vi "skippable_AlliGator SS2 Dataset Load Option Dialog.vi"(8 "Error In":errorcluster) -> (0 "Error Out":errorcluster, 3 "SS2 8-bit Frame Selection":T1 caption="SS2 Frame Selection")   [LabVIEW 2021, in "AlliGator Files.lvlib"]
doc: "Skippable dialog to determine which 8-bit frame to load out of the 4 constituting a 10-bit dataset."
uses:
  AlliGator/AlliGator Files.lvlib
  SwissSPAD 8-bit Frames Read.ctl
  <vilib>/Utility/error.llb/Error Cluster From Error Code.vi
  <vilib>/ErrorRing/Error Ring.xnode
  AlliGator/AlliGator GUI.lvlib
  SwissSPAD.lvlib
panel:
  in  "Cancel":bool
  in  "SS2 Frame Selection":T1
  in  "OK":bool
  in  "Do not show this dialog again":bool
  out "Displayed Message":string="Select which 8-bit component to include in the final dataset:"
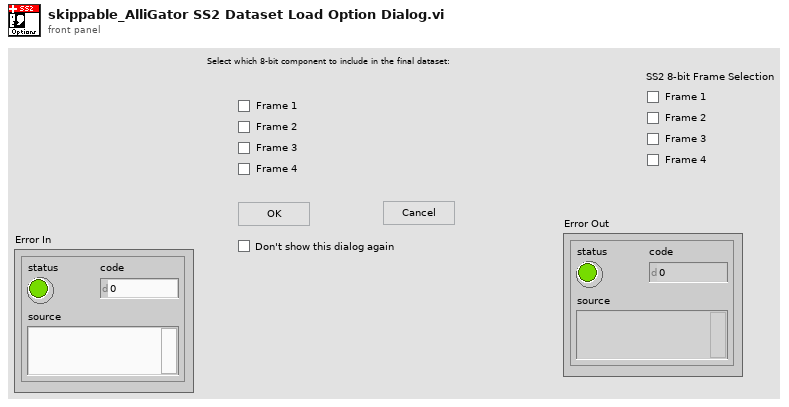
[diagram p1: front panel]
types:
  T1 = typedef "SwissSPAD.lvlib/SwissSPAD 8-bit Frames Read.ctl" = cluster{"Frame 1":bool, "Frame 2":bool, "Frame 3":bool, "Frame 4":bool}
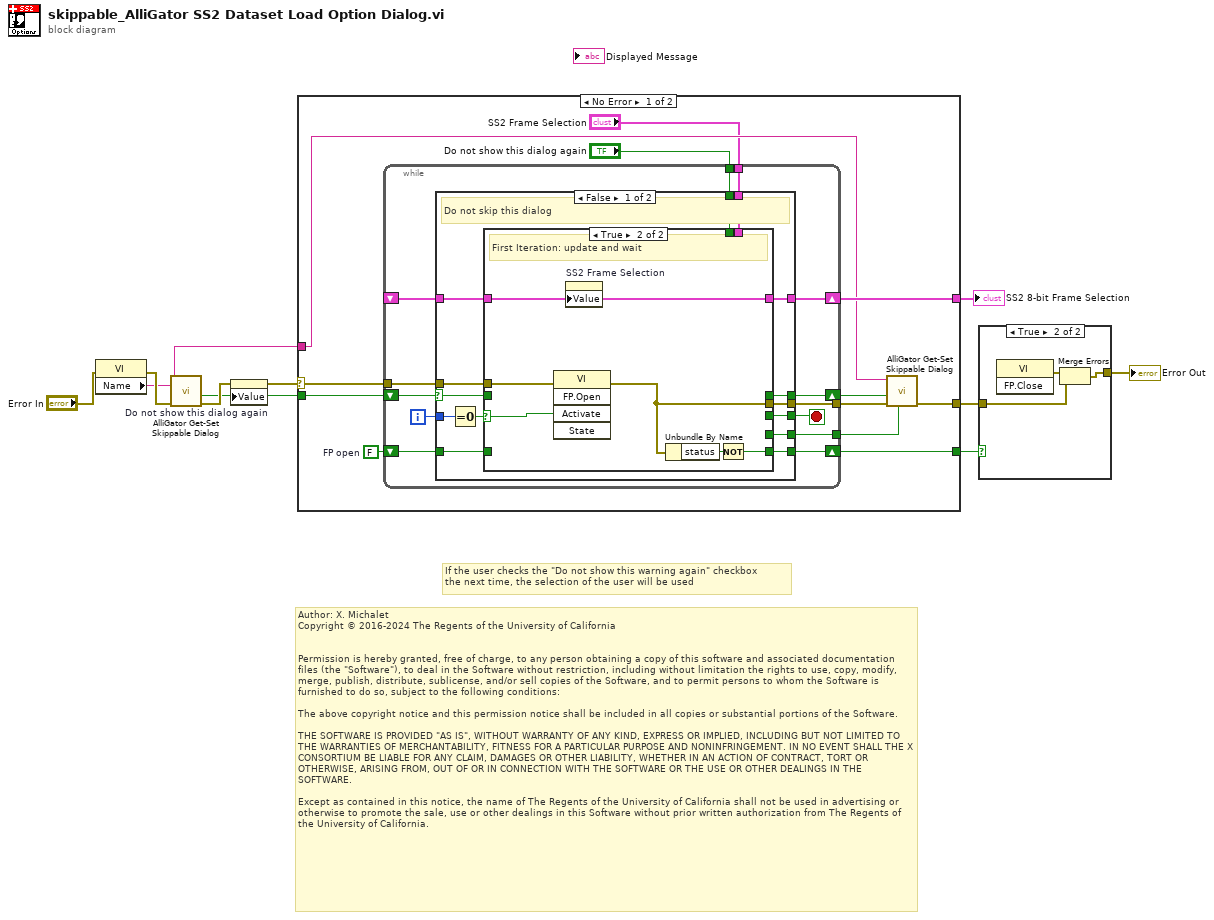
[diagram p0: block diagram]
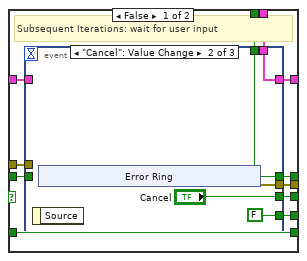
[diagram p3: hidden frame]
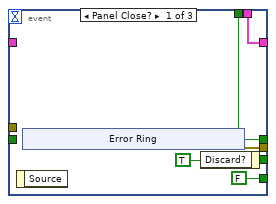
[diagram p4: hidden frame]
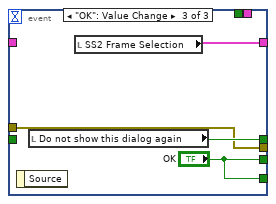
[diagram p5: hidden frame]
diagram:
  # "Author: X. Michalet\nCopyright © 2016-2024 The Regents of the University of California\n \n\nPermission is hereby granted, free of charge, to any person obtaining a copy of this software and associated documentation files (the \"Software\"), to deal in the Software without restriction, including without limitation the rights to use, copy, modify, merge, publish, distribute, sublicense, and/or sell copies of the Software, and to permit persons to whom the Software is furnished to do so, subject to the following conditions:\n\nThe above copyright notice and this permission notice shall be included in all copies or substantial portions of the Software.\n\nTHE SOFTWARE IS PROVIDED \"AS IS\", WITHOUT WARRANTY OF ANY KIND, EXPRESS OR IMPLIED, INCLUDING BUT NOT LIMITED TO THE WARRANTIES OF MERCHANTABILITY, FITNESS FOR A PARTICULAR PURPOSE AND NONINFRINGEMENT. IN NO EVENT SHALL THE X CONSORTIUM BE LIABLE FOR ANY CLAIM, DAMAGES OR OTHER LIABILITY, WHETHER IN AN ACTION OF CONTRACT, TORT OR OTHERWISE, ARISING FROM, OUT OF OR IN CONNECTION WITH THE SOFTWARE OR THE USE OR OTHER DEALINGS IN THE SOFTWARE.\n\nExcept as contained in this notice, the name of The Regents of the University of California shall not be used in advertising or otherwise to promote the sale, use or other dealings in this Software without prior written authorization from The Regents of the University of California."
  # "If the user checks the \"Do not show this warning again\" checkbox\nthe next time, the selection of the user will be used"
  n1 = property class="VI"(error in="Error In") -> (error out=w8:errorcluster, "Name"=w7:string)  [unwired: 1 in, 1 out]
  n2 = call "AlliGator Get-Set Skippable Dialog.vi"("Error In"=w8, "Dialog Window VI Name"=w7) -> ("Error Out"=w4:errorcluster, "Is skipped (out)"=w3:bool)  [unwired: 8 in]
  n3 = property on="Do not show this dialog again" class="Bool (strict)"(error in=w4, "Value"=w3) -> (error out=w2:errorcluster)  [unwired: 1 in, 1 out]
  n4 = case shown="No Error" w2 {
    selector: w2 -> [w14 w93]
    tunnel: [w22 _] -> w10
    tunnel: w3 -> [w21 _]
    tunnel: w7 -> [w18 _]
    tunnel: [w17 w93] -> w6
    tunnel: [w11 _] -> w1
    frame No Error {
      w12 = FALSE  # FP open
      n5 = while {
        shift-right: [w35] -> w19
        shift-left: w21 -> [w33]
        shift-right: [w30] -> w22
        shift-left: _ -> [w31]
        tunnel: "Do not show this dialog again" -> [w29]
        tunnel: [w28] -> w16
        tunnel: "SS2 Frame Selection" -> [w27]
        tunnel: w14 -> [w26]
        tunnel: [w25] -> w13
        shift-right: [w24] -> w11
        shift-left: w12 -> [w23]
        i -> [w34]
        stop <- w32 stop-if-true
        n6 = case shown="False" w33 {
          selector: w33 -> [w47 w91]
          tunnel: [w49 w91] -> w35
          tunnel: w34 -> [w48 _]
          tunnel: [w46 w91] -> w32
          tunnel: w31 -> [w45 w92]
          tunnel: [w44 w92] -> w30
          tunnel: w29 -> [w43 _]
          tunnel: [w41 w91] -> w28
          tunnel: w27 -> [w40 _]
          tunnel: w26 -> [w39 w90]
          tunnel: [w38 w90] -> w25
          tunnel: [w37 w89] -> w24
          tunnel: w23 -> [w36 w89]
          frame False {
            # "Do not skip this dialog"
            n7 = Equal To 0?(x=w48) -> (x = 0?=w42:bool)
            n8 = case shown="True" w42 {
              selector: w42 -> [_ w88]
              tunnel: [w60 _] -> w46
              tunnel: [w59 _] -> w49
              tunnel: w47 -> [w58 _]
              tunnel: w45 -> [w57 w87]
              tunnel: [w56 w87] -> w44
              tunnel: w43 -> [w55 _]
              tunnel: [w54 _] -> w41
              tunnel: w40 -> [w53 _]
              tunnel: w39 -> [w52 w86]
              tunnel: [w51 w85] -> w38
              tunnel: [w50 w83] -> w37
              tunnel: w36 -> [w50 _]
              frame False {
                # "Subsequent Iterations: wait for user input"
                n9 = event shown="[1] \"Cancel\": Value Change" {
                  selector: _ -> [_ _ _]
                  dyn-events: _ -> [_ _ _]
                  timeout: _ -> [_ _ _]
                  tunnel: [w65 "Cancel" "OK"] -> w60
                  tunnel: [w64 w74 w82] -> w59
                  tunnel: w58 -> [_ _ _]
                  tunnel: w57 -> [_ _ _]
                  tunnel: [w62 w72 w81] -> w56
                  tunnel: w55 -> [w64 w74 _]
                  tunnel: [FALSE ("Discard?") FALSE ("Discard?") "OK"] -> w54
                  tunnel: w53 -> [w62 w72 _]
                  tunnel: w52 -> [_ _ w79]
                  tunnel: [w61 w71 w79] -> w51
                  event Panel Close? {
                    w65 = TRUE ("Discard?")
                    n10 = event-data() -> ()  [unwired: 1 in, 1 out]
                    n11 = xnode "Error Ring"() -> ("error out"=w61:errorcluster)
                    n12 = event-data("Discard?"=w65) -> ()  [unwired: 1 in, 1 out]
                  }
                  event "Cancel": Value Change {
                    n13 = event-data() -> ()  [unwired: 1 in, 1 out]
                    n14 = xnode "Error Ring"() -> ("error out"=w71:errorcluster)
                  }
                  event "OK": Value Change {
                    n15 = event-data() -> ()  [unwired: 1 in, 1 out]
                    n16 = local read "Do not show this dialog again"() -> (w82:bool)
                    n17 = local read "SS2 Frame Selection"() -> (w81:T1)
                  }
                }
              }
              frame True {
                # "First Iteration: update and wait"
                n18 = invoke class="VI" method="FP.Open"(error in=w86, "Activate"=w88) -> (error out=w85:errorcluster)  [unwired: 3 in, 4 out]
                n19 = property on="SS2 Frame Selection" class="Clust (strict)"("Value"=w87) -> ()  [unwired: 2 in, 2 out]
                n20 = Unbundle By Name(w85) -> ("status"=w84:bool)
                n21 = Not(x=w84) -> (.not. x?=w83:bool)
              }
            }
          }
          frame True {
            # "skip this dialog"
          }
        }
      }
      n22 = call "AlliGator Get-Set Skippable Dialog.vi"("Set/Get (F)"=w16, "Error In"=w13, "Is skipped (in)"=w19, "Dialog Window VI Name"=w18) -> ("Error Out"=w17:errorcluster)  [unwired: 6 in, 1 out]
    }
    frame Error {
    }
  }
  "SS2 8-bit Frame Selection" <- w10
  n23 = case shown="True" w1 {
    tunnel: w6 -> [w94 w95]
    tunnel: [w94 w96] -> w5
    frame False {
    }
    frame True {
      n24 = invoke class="VI" method="FP.Close"() -> (error out=w97:errorcluster)  [unwired: 3 in, 2 out]
      n25 = Merge Errors(w97, w95) -> (w96:errorcluster)
    }
  }
  "Error Out" <- w5
